vi "Write Multiple Samples.vi"(0 "TDMS In":refnum<k34>, 5 "Input Vector":sgl[][](array[numeric]), 7 "Output Vector":sgl[][](array[numeric]), 11 "Error In":errorcluster) -> (4 "TDMS Out":refnum<k34>, 15 "Error Out":errorcluster)   [LabVIEW 2015, in "Teaching File.lvlib"]
doc: "Write multiple teaching samples to the TDMS file. Columns represent seperate IO and the rows represent seperate samples.\n\nThe group names used will be <b>Input_Data</b> and <b>Output_Data</b>. Channels will correspond to the index of IO in the teaching sample. If the group or the channels do not exist in TDMS, they will be created.\n\nIf the lengths of the wired samples are not matching the samples already in the file, return error 7123."
uses:
  Teaching File.lvlib
  <vilib>/ErrorRing/Error Ring.xnode
  <vilib>/Utility/error.llb/Error Cluster From Error Code.vi
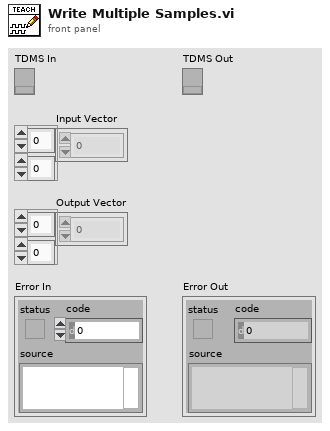
[diagram p1: front panel]
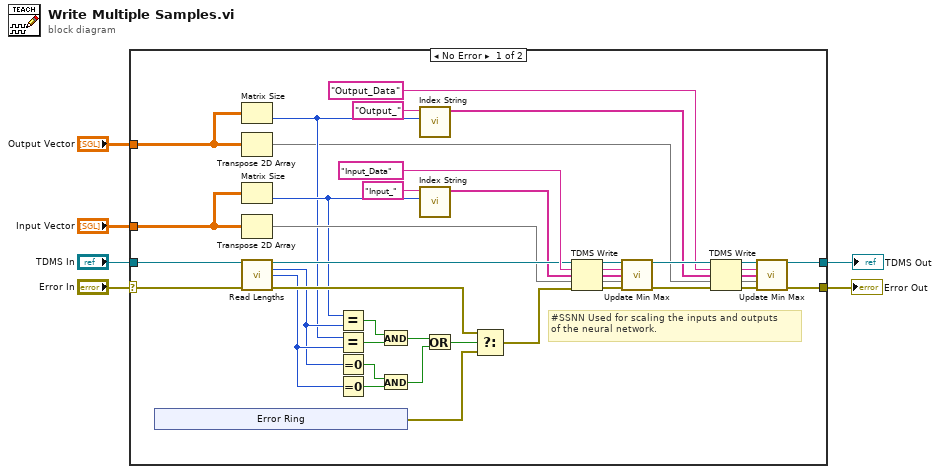
[diagram p0: block diagram]
diagram:
  n1 = case shown="No Error" "Error In" {
    selector: "Error In" -> [w8 w52]
    tunnel: "Output Vector" -> [w40 _]
    tunnel: "Input Vector" -> [w39 _]
    tunnel: "TDMS In" -> [w38 w51]
    tunnel: [w16 w51] -> w3
    tunnel: [w15 w52] -> w2
    frame No Error {
      # "#SSNN Used for scaling the inputs and outputs\nof the neural network."
      n2 = xnode "Error Ring"() -> ("error out"=w28:errorcluster)
      n3 = Matrix Size(0:w40) -> (2:w11:i32)  [unwired: 1 out]
      n4 = Transpose 2D Array(2D array=w40) -> (transposed array=w7:sgl[][])
      n5 = Matrix Size(0:w39) -> (2:w13:i32)  [unwired: 1 out]
      n6 = Transpose 2D Array(2D array=w39) -> (transposed array=w24:sgl[][])
      n7 = call "Read Lengths.vi"("TDMS In"=w38, "Error In"=w8) -> ("TDMS Out"=w37:refnum<k34>, "# Inputs"=w25:i32, "# Outputs"=w26:i32, "Error Out"=w29:errorcluster)  [unwired: 9 in, 1 out]
      n8 = Equal?(x=w13, y=w25) -> (x = y?=w35:bool)
      n9 = Equal?(x=w11, y=w26) -> (x = y?=w36:bool)
      n10 = Equal To 0?(x=w25) -> (x = 0?=w34:bool)
      n11 = Equal To 0?(x=w26) -> (x = 0?=w33:bool)
      n12 = And(x=w35, y=w36) -> (x .and. y?=w32:bool)
      n13 = And(x=w34, y=w33) -> (x .and. y?=w31:bool)
      n14 = call "Index String.vi"("N"=w11, "String"="Output_" ("group name in")) -> ("Indexed Strings"=w9:string[])  [unwired: 9 in]
      n15 = call "Index String.vi"("N"=w13, "String"="Input_" ("group name in")) -> ("Indexed Strings"=w12:string[])  [unwired: 9 in]
      n16 = Or(x=w32, y=w31) -> (x .or. y?=w30:bool)
      n17 = Select(t=w29, s=w30, f=w28) -> (s? t:f=w27:errorcluster)
      n18 = TDMS Write(0:w37, 5:"Input_Data" ("group name in"), 7:w12, 9:w24, 11:w27) -> (4:w43:refnum<k34>, 6:w42:string, 8:w41:string[], 15:w44:errorcluster)  [unwired: 1 in]
      n19 = call "Update Min Max.vi"("TDMS In"=w43, "Group"=w42, "Channels"=w41, "Value/Channel"=w24, "Error In"=w44) -> ("TDMS Out"=w19:refnum<k34>, "Error Out"=w18:errorcluster)  [unwired: 9 in]
      n20 = TDMS Write(0:w19, 5:"Output_Data" ("group name in"), 7:w9, 9:w7, 11:w18) -> (4:w21:refnum<k34>, 6:w22:string, 8:w23:string[], 15:w20:errorcluster)  [unwired: 1 in]
      n21 = call "Update Min Max.vi"("TDMS In"=w21, "Group"=w22, "Channels"=w23, "Value/Channel"=w7, "Error In"=w20) -> ("TDMS Out"=w16:refnum<k34>, "Error Out"=w15:errorcluster)  [unwired: 9 in]
    }
    frame Error {
    }
  }
  "Error Out" <- w2
  "TDMS Out" <- w3
